vi "Check for SR List File.vi"(8 "error in":errorcluster) -> (0 "error out":errorcluster, 2 "list exists":bool)   [LabVIEW 2018]
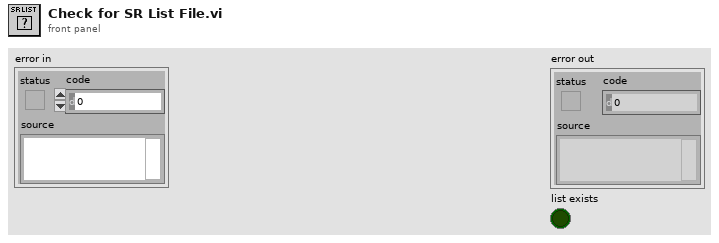
[diagram p1: front panel]
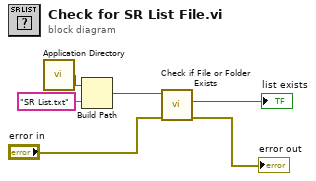
[diagram p0: block diagram]
diagram:
  n1 = call <vilib>:"Application Directory.vi"() -> ("Application Directory"=w4:path)
  n2 = Build Path(base path=w4, name or relative path="SR List.txt") -> (appended path=w6:path)
  n3 = call <vilib>:"Check if File or Folder Exists.vi"("error in (no error)"="error in", "path"=w6) -> ("error out"=→"error out":errorcluster, "file or folder exists?"=→"list exists":bool)  [unwired: 7 in, 1 out]
